vi "Sort_Dust_Array.vi"(1 "Order by...":T1(ring), 2 "Array In":T2[](array[typedef])) -> (0 "Array out":T2[](array[typedef]))   [LabVIEW 2013]
doc: "Takes a given array of dust_type elements, and returns the same array, ordered by the given column. Ordering by \"dust_name\" will order first by \"dust_name\", second by the \"dust_type\", and third by \"batch_no\"."
uses:
  User Interface/Controls/Dust_list.ctl
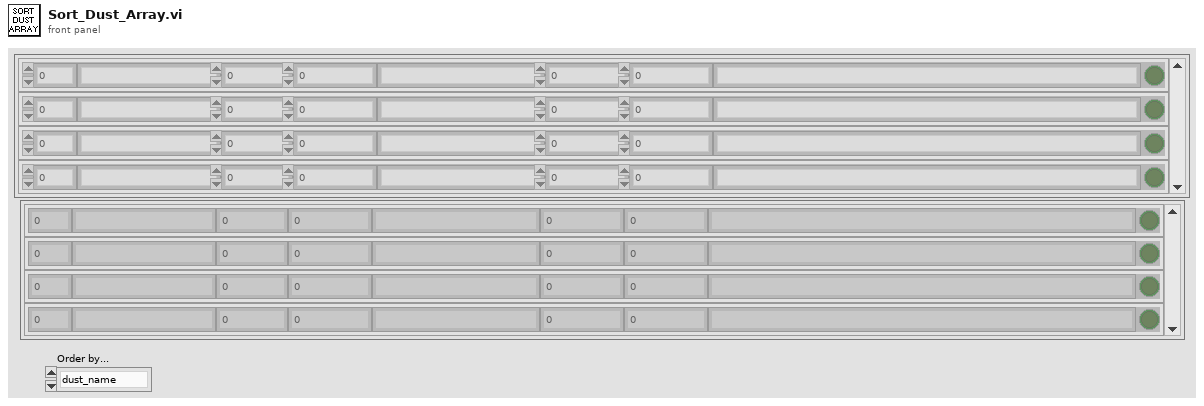
[diagram p1: front panel]
types:
  T1 = enum16{"dust_name", "dust_density", "source_weight", "bottle_weight", "dust_weight"}
  T2 = typedef "Dust_list.ctl" = cluster{"id_dust_type":i32, "dust_name":string, "dust_type":i32, "batch_no":i32, "dust_density":dbl, "source_weight":dbl, "size":string, "bottle_weight":dbl, "dust_mass":dbl, "comments":string, "Shoots?":bool}
  T3 = cluster{"dust_name":string, "dust_type":i32, "batch_no":i32, "index":i32}
  T4 = cluster{"dust_name":string, "dust_type":i32, "batch_no":i32, "index":i32}[]
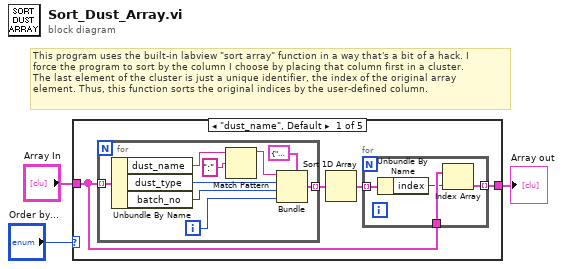
[diagram p0: block diagram]
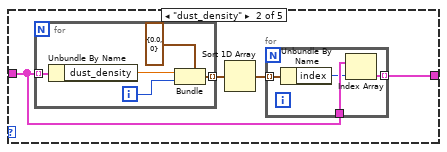
[diagram p2: hidden frame]
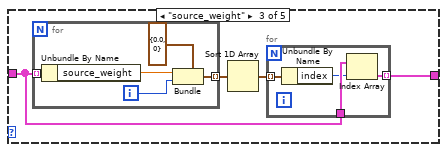
[diagram p3: hidden frame]
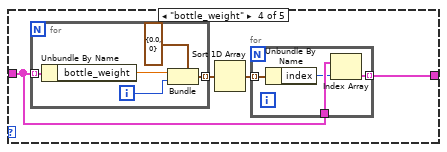
[diagram p4: hidden frame]
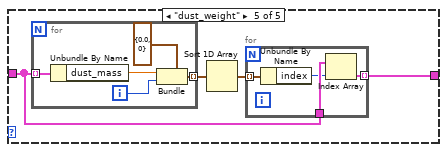
[diagram p5: hidden frame]
diagram:
  # "This program uses the built-in labview \"sort array\" function in a way that's a bit of a hack. I\nforce the program to sort by the column I choose by placing that column first in a cluster.\nThe last element of the cluster is just a unique identifier, the index of the original array\nelement. Thus, this function sorts the original indices by the user-defined column."
  n1 = case shown="\"dust_name\", Default" "Order by..." {
    tunnel: "Array In" -> [w6 w23 w36 w49 w62]
    tunnel: [w4 w21 w34 w47 w60] -> w1
    frame "dust_name", Default {
      n2 = for {
        tunnel: w6 -> [w20] mode=indexing
        tunnel: [w19] -> w5 mode=indexing
        i -> [w17]
        n3 = Unbundle By Name(w20) -> ("dust_name"=w14:string, "dust_type"=w16:i32, "batch_no"=w15:i32)
        n4 = Match Pattern(string=w14, regular expression=":") -> (before substring=w12:string)  [unwired: 1 in, 3 out]
        n5 = Bundle(cluster=T3 {"dust_name"="", "dust_type"=0, "batch_no"=0, "index"=0}, "dust_name"=w12, "dust_type"=w16, "batch_no"=w15, "index"=w17) -> (w19:T3)
      }
      n6 = Sort 1D Array(array=w5) -> (sorted array=w7:T4)
      n7 = for {
        tunnel: w7 -> [w11] mode=indexing
        tunnel: w6 -> [w10]
        tunnel: [w8] -> w4 mode=indexing
        n8 = Unbundle By Name(w11) -> ("index"=w9:i32)
        n9 = Index Array(array=w10, index=w9) -> (element=w8:T2)
      }
    }
    frame "dust_density" {
      n10 = for {
        tunnel: w23 -> [w33] mode=indexing
        tunnel: [w31] -> w22 mode=indexing
        i -> [w30]
        n11 = Unbundle By Name(w33) -> ("dust_density"=w32:dbl)
        n12 = Bundle(cluster=cluster{"dust_name":dbl, "index":i32} {"dust_name"=0.0, "index"=0}, "dust_name"=w32, "index"=w30) -> (w31:cluster{"dust_name":dbl, "index":i32})
      }
      n13 = Sort 1D Array(array=w22) -> (sorted array=w24:cluster{"dust_name":dbl, "index":i32}[])
      n14 = for {
        tunnel: w24 -> [w28] mode=indexing
        tunnel: w23 -> [w27]
        tunnel: [w25] -> w21 mode=indexing
        n15 = Unbundle By Name(w28) -> ("index"=w26:i32)
        n16 = Index Array(array=w27, index=w26) -> (element=w25:T2)
      }
    }
    frame "source_weight" {
      n17 = for {
        tunnel: w36 -> [w46] mode=indexing
        tunnel: [w44] -> w35 mode=indexing
        i -> [w43]
        n18 = Unbundle By Name(w46) -> ("source_weight"=w45:dbl)
        n19 = Bundle(cluster=cluster{"dust_name":dbl, "index":i32} {"dust_name"=0.0, "index"=0}, "dust_name"=w45, "index"=w43) -> (w44:cluster{"dust_name":dbl, "index":i32})
      }
      n20 = Sort 1D Array(array=w35) -> (sorted array=w37:cluster{"dust_name":dbl, "index":i32}[])
      n21 = for {
        tunnel: w37 -> [w41] mode=indexing
        tunnel: w36 -> [w40]
        tunnel: [w38] -> w34 mode=indexing
        n22 = Unbundle By Name(w41) -> ("index"=w39:i32)
        n23 = Index Array(array=w40, index=w39) -> (element=w38:T2)
      }
    }
    frame "bottle_weight" {
      n24 = for {
        tunnel: w49 -> [w59] mode=indexing
        tunnel: [w57] -> w48 mode=indexing
        i -> [w56]
        n25 = Unbundle By Name(w59) -> ("bottle_weight"=w58:dbl)
        n26 = Bundle(cluster=cluster{"dust_name":dbl, "index":i32} {"dust_name"=0.0, "index"=0}, "dust_name"=w58, "index"=w56) -> (w57:cluster{"dust_name":dbl, "index":i32})
      }
      n27 = Sort 1D Array(array=w48) -> (sorted array=w50:cluster{"dust_name":dbl, "index":i32}[])
      n28 = for {
        tunnel: w50 -> [w54] mode=indexing
        tunnel: w49 -> [w53]
        tunnel: [w51] -> w47 mode=indexing
        n29 = Unbundle By Name(w54) -> ("index"=w52:i32)
        n30 = Index Array(array=w53, index=w52) -> (element=w51:T2)
      }
    }
    frame "dust_weight" {
      n31 = for {
        tunnel: w62 -> [w72] mode=indexing
        tunnel: [w70] -> w61 mode=indexing
        i -> [w69]
        n32 = Unbundle By Name(w72) -> ("dust_mass"=w71:dbl)
        n33 = Bundle(cluster=cluster{"dust_name":dbl, "index":i32} {"dust_name"=0.0, "index"=0}, "dust_name"=w71, "index"=w69) -> (w70:cluster{"dust_name":dbl, "index":i32})
      }
      n34 = Sort 1D Array(array=w61) -> (sorted array=w63:cluster{"dust_name":dbl, "index":i32}[])
      n35 = for {
        tunnel: w63 -> [w67] mode=indexing
        tunnel: w62 -> [w66]
        tunnel: [w64] -> w60 mode=indexing
        n36 = Unbundle By Name(w67) -> ("index"=w65:i32)
        n37 = Index Array(array=w66, index=w65) -> (element=w64:T2)
      }
    }
  }
  "Array out" <- w1
